vi "Split GB Count.vi"(11 "Split GB":dbl) -> (2 "Split":bool, 3 "Split Count":i32)   [LabVIEW 2020, in "VolatusData.lvlib" / "Data Logger Module.lvclass"]
uses:
  Data Logger Module.lvclass
  Data Logger Module.lvclass/Data Logger Module.ctl
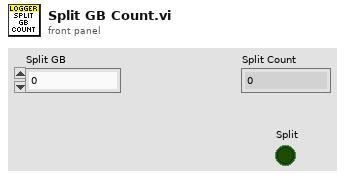
[diagram p1: front panel]
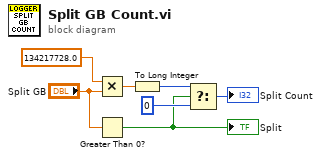
[diagram p0: block diagram]
diagram:
  n1 = Multiply(x=134217728.0, y="Split GB") -> (x*y=w5:dbl)
  n2 = Greater Than 0?(x="Split GB") -> (x > 0?=w2:bool)
  "Split" <- w2
  n3 = To Long Integer(number=w5) -> (32bit integer=w4:i32)
  n4 = Select(t=w4, s=w2, f=0 ("t")) -> (s? t:f=→"Split Count":i32)
